vi "Send Message.vi"(8 "error in (no error)":errorcluster, 10 "Architecture.lvlib:Message.lvclass":refnum<class "Message.lvclass">, 11 "Queue in":refnum<class "Queue.lvclass">) -> (0 "error out":errorcluster, 3 "Queue out":refnum<class "Queue.lvclass">)   [LabVIEW 2013, in "Architecture.lvlib" / "Queue.lvclass"]
uses:
  Queue.lvclass
  Message.lvclass
  Queue.lvclass/Queue.ctl
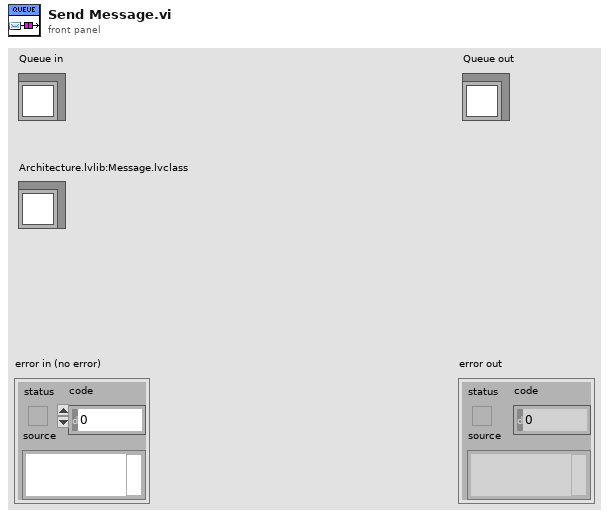
[diagram p1: front panel]
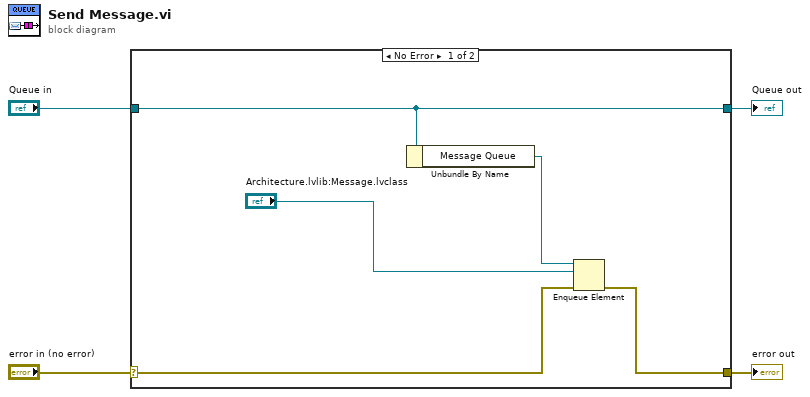
[diagram p0: block diagram]
diagram:
  n1 = case shown="No Error" "error in (no error)" {
    selector: "error in (no error)" -> [w6 w11]
    tunnel: [w5 w11] -> w3
    tunnel: [w9 w10] -> w1
    tunnel: "Queue in" -> [w9 w10]
    frame No Error {
      n2 = Unbundle By Name(w9) -> ("Message Queue"=w8:refnum<queue>)
      n3 = Enqueue Element(queue=w8, element="Architecture.lvlib:Message.lvclass", error in (no error)=w6) -> (error out=w5:errorcluster)  [unwired: 1 in, 2 out]
    }
    frame Error {
    }
  }
  "error out" <- w3
  "Queue out" <- w1
